vi "Load Existing Selected XNET Signals.vi"(6 "Disabled? (False)":bool, 7 "Symbol Index (38)":i32=38, 8 "error in (no error)":errorcluster, 9 "Parent":string, 10 "Node Ptr":u64 format="%.0x", 11 "Tree":refnum<vi>) -> (0 "error out":errorcluster, 2 "Node Ptr":u64 format="%.0x", 3 "Tree Out":refnum<vi>)   [LabVIEW 2015, in "J1939 Addon System Explorer.lvlib"]
uses:
  J1939 Addon System Explorer.lvlib
  Shared/SubVIs/Constants.vi
  <vilib>/NI VeriStand/Custom Device API/Custom Device API.lvlib
  Shared/J1939 Addon Shared.lvlib
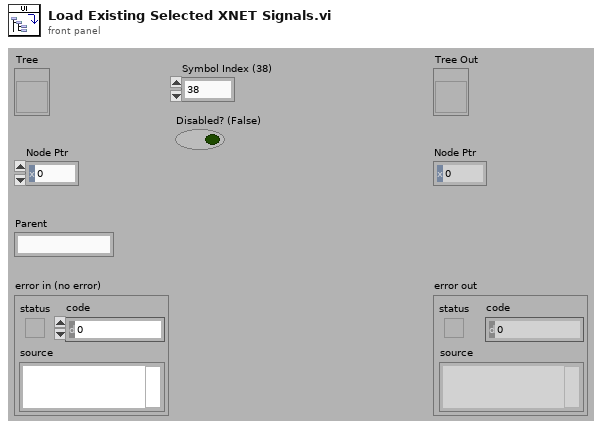
[diagram p1: front panel]
types:
  T1 = typedef "Custom Device API.lvlib/Custom Device Item Ref.ctl" = u64
  T2 = typedef "Custom Device API.lvlib/Custom Device Item Info.ctl" = cluster{"Name":string, "Is Channel":bool, "GUID":string, "Is Waveform":bool}
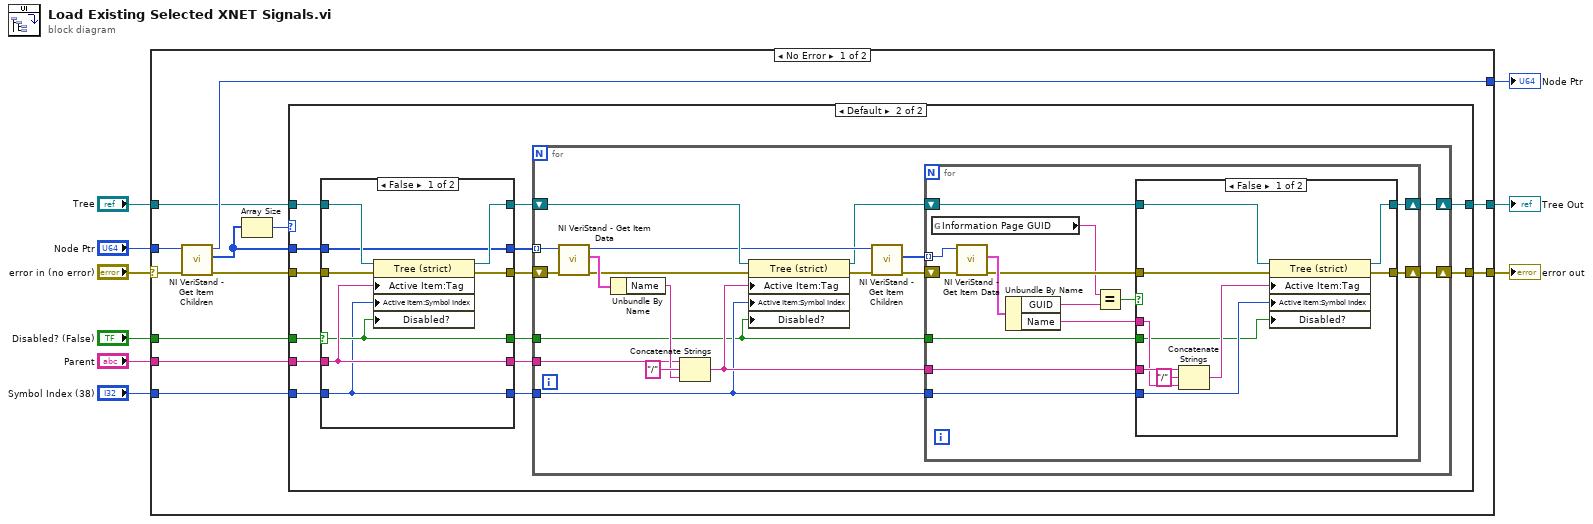
[diagram p0: block diagram]
diagram:
  n1 = case shown="No Error" "error in (no error)" {
    selector: "error in (no error)" -> [w21 w98]
    tunnel: [w19 w98] -> w8
    tunnel: "Node Ptr" -> [w20 w96]
    tunnel: "Tree" -> [w15 w97]
    tunnel: [w18 w97] -> w5
    tunnel: "Parent" -> [w14 _]
    tunnel: [w17 w96] -> w3
    tunnel: "Symbol Index (38)" -> [w11 _]
    tunnel: "Disabled? (False)" -> [w10 _]
    frame No Error {
      n2 = call <vilib>:"NI VeriStand - Get Item Children.vi"("error in (no error)"=w21, "Item Ref in"=w20) -> ("error out"=w16:errorcluster, "Child Refs"=w13:T1[], "Item Ref out"=w17:T1)  [unwired: 6 in, 1 out]
      n3 = Array Size(array=w13) -> (size(s)=w12:i32)
      n4 = case shown="Default" w12 {
        tunnel: [w23 w37] -> w19
        tunnel: [w22 w36] -> w18
        tunnel: w16 -> [w23 w35]
        tunnel: w15 -> [w22 w33]
        tunnel: w14 -> [_ w31]
        tunnel: w13 -> [_ w25]
        tunnel: w11 -> [_ w30]
        tunnel: w10 -> [_ w29]
        frame 0 {
        }
        frame Default {
          n5 = case shown="False" w29 {
            selector: w29 -> [w40 w49]
            tunnel: w35 -> [w45 w50]
            tunnel: [w44 w50] -> w34
            tunnel: w33 -> [w43 w51]
            tunnel: [w42 w51] -> w32
            tunnel: w31 -> [w41 w48]
            tunnel: w30 -> [w38 w46]
            tunnel: [w40 w49] -> w28
            tunnel: [w41 w48] -> w27
            tunnel: [w39 w47] -> w26
            tunnel: w25 -> [w39 w47]
            tunnel: [w38 w46] -> w24
            frame False {
              n6 = property class="Tree (strict)"(reference=w43, error in=w45, "Active Item:Tag"=w41, "Active Item:Symbol Index"=w38, "Disabled?"=w40) -> (reference out=w42:refnum<vi>, error out=w44:errorcluster)
            }
            frame True {
            }
          }
          n7 = for {
            tunnel: w26 -> [w68] mode=indexing
            shift-right: [w59] -> w36
            shift-left: w32 -> [w64]
            shift-right: [w58] -> w37
            shift-left: w34 -> [w69]
            tunnel: w27 -> [w54]
            tunnel: w24 -> [w53]
            tunnel: w28 -> [w52]
            n8 = call <vilib>:"NI VeriStand - Get Item Data.vi"("error in (no error)"=w69, "Item Ref in"=w68) -> ("error out"=w66:errorcluster, "Item Info"=w67:T2, "Item Ref out"=w63:T1)  [unwired: 6 in, 1 out]
            n9 = Unbundle By Name(w67) -> ("Name"=w56:string)
            n10 = Concatenate Strings(w54, "/" ("string"), w56) -> (w55:string)
            n11 = property class="Tree (strict)"(reference=w64, error in=w66, "Active Item:Tag"=w55, "Active Item:Symbol Index"=w53, "Disabled?"=w52) -> (reference out=w60:refnum<vi>, error out=w65:errorcluster)
            n12 = call <vilib>:"NI VeriStand - Get Item Children.vi"("error in (no error)"=w65, "Item Ref in"=w63) -> ("error out"=w62:errorcluster, "Child Refs"=w61:T1[])  [unwired: 6 in, 2 out]
            n13 = for {
              tunnel: w61 -> [w82] mode=indexing
              shift-right: [w78] -> w59
              shift-left: w60 -> [w79]
              shift-right: [w77] -> w58
              shift-left: w62 -> [w83]
              tunnel: w55 -> [w76]
              tunnel: w53 -> [w74]
              tunnel: w52 -> [w73]
              n14 = global read "Constants.vi" "Information Page GUID"() -> (w71:string)
              n15 = call <vilib>:"NI VeriStand - Get Item Data.vi"("error in (no error)"=w83, "Item Ref in"=w82) -> ("error out"=w80:errorcluster, "Item Info"=w81:T2)  [unwired: 6 in, 2 out]
              n16 = Unbundle By Name(w81) -> ("GUID"=w72:string, "Name"=w75:string)
              n17 = Equal?(x=w71, y=w72) -> (x = y?=w70:bool)
              n18 = case shown="False" w70 {
                tunnel: w80 -> [w93 w94]
                tunnel: w79 -> [w92 w95]
                tunnel: [w91 w95] -> w78
                tunnel: [w90 w94] -> w77
                tunnel: w76 -> [w88 _]
                tunnel: w75 -> [w87 _]
                tunnel: w74 -> [w85 _]
                tunnel: w73 -> [w84 _]
                frame False {
                  n19 = Concatenate Strings(w88, "/" ("string"), w87) -> (w86:string)
                  n20 = property class="Tree (strict)"(reference=w92, error in=w93, "Active Item:Tag"=w86, "Active Item:Symbol Index"=w85, "Disabled?"=w84) -> (reference out=w91:refnum<vi>, error out=w90:errorcluster)
                }
                frame True {
                }
              }
            }
          }
        }
      }
    }
    frame Error {
    }
  }
  "error out" <- w8
  "Tree Out" <- w5
  "Node Ptr" <- w3
